vi "Load Parameters From XML.vi"() -> (0 "error out":errorcluster, 2 "dynamic parameters":cluster{"Thumb":T1, "Middle":T1, "Index":T1}, 3 "kinematic parameters":T4)   [LabVIEW 2011, in "MF3.lvclass"]
uses:
  MF3.lvclass
  <vilib>/robotics/Kinematics/Link/Joint Type.ctl
  Controls/5-bar Side.ctl
  Controls/Dynamic Parameters.ctl
  <vilib>/NI/GXML/_subVIs/GXML SearchParser/Search Parser.vi
  <vilib>/NI/GXML/GXML.lvlib
  <vilib>/robotics/Kinematics/Link/NI_Robotics_Link.lvclass
panel:
  out "file path":path
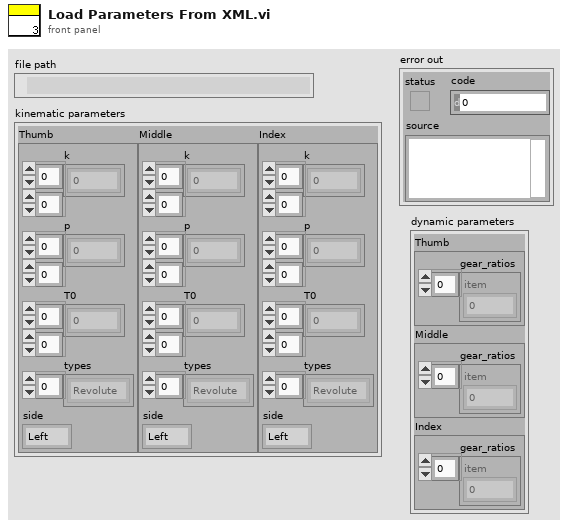
[diagram p1: front panel]
types:
  T1 = typedef "Dynamic Parameters.ctl" = cluster{"gear_ratios":sgl[]}
  T2 = typedef "NI_Robotics_Link.lvclass/Joint Type.ctl" = enum16{"Revolute", "Prismatic"}
  T3 = typedef "5-bar Side.ctl" = enum16{"Left", "Right"}
  T4 = cluster{"Thumb":cluster{"k":sgl[][], "p":sgl[][], "T0":sgl[][], "types":T2[], "side":T3}, "Middle":cluster{"k":sgl[][], "p":sgl[][], "T0":sgl[][], "types":T2[], "side":T3}, "Index":cluster{"k":sgl[][], "p":sgl[][], "T0":sgl[][], "types":T2[], "side":T3}}
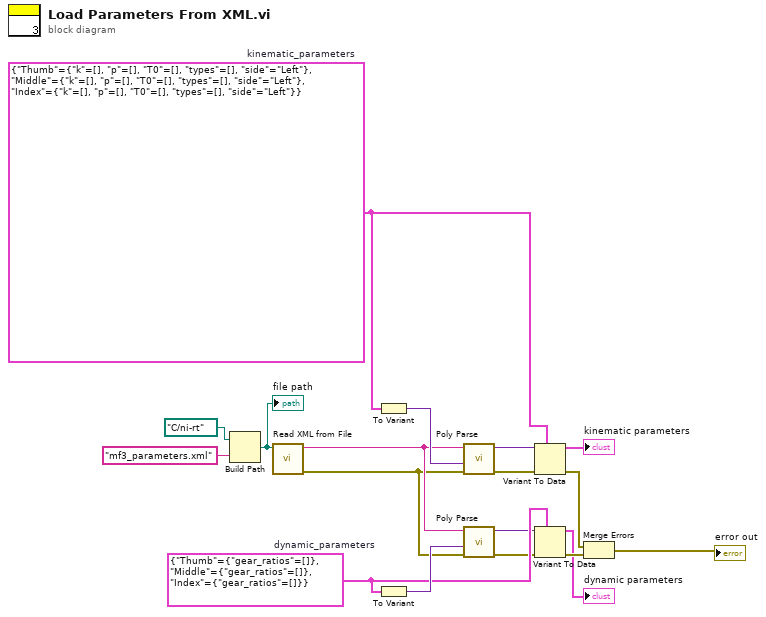
[diagram p0: block diagram]
diagram:
  w6 = cluster{"Thumb":T1, "Middle":T1, "Index":T1} {"Thumb"={"gear_ratios"=[]}, "Middle"={"gear_ratios"=[]}, "Index"={"gear_ratios"=[]}}  # dynamic_parameters
  w13 = T4 {"Thumb"={"k"=[], "p"=[], "T0"=[], "types"=[], "side"=enum."Left"}, "Middle"={"k"=[], "p"=[], "T0"=[], "types"=[], "side"=enum."Left"}, "Index"={"k"=[], "p"=[], "T0"=[], "types"=[], "side"=enum."Left"}}  # kinematic_parameters
  n1 = Build Path(base path=path "C:/ni-rt", name or relative path="mf3_parameters.xml") -> (appended path=w16:path)
  "file path" <- w16
  n2 = call <vilib>:"Read XML from File.vi"("XML File Path"=w16) -> ("error out"=w9:errorcluster, "XML String Out"=w10:string)  [unwired: 9 in]
  n3 = To Variant(anything=w13) -> (Variant=w15:variant)
  n4 = To Variant(anything=w6) -> (Variant=w11:variant)
  n5 = call-poly <vilib>:"Poly Parse.vi"("error in"=w9, "TypeDesc"=w15, "XML String In"=w10) -> ("error out"=w8:errorcluster, "Parsed Data"=w14:variant)  [unwired: 7 in]
  n6 = call-poly <vilib>:"Poly Parse.vi"("error in"=w9, "TypeDesc"=w11, "XML String In"=w10) -> ("error out"=w4:errorcluster, "Parsed Data"=w5:variant)  [unwired: 7 in]
  n7 = Variant To Data(error in=w8, type=w13, Variant=w14) -> (data=→"kinematic parameters":T4, error out=w7:errorcluster)
  n8 = Variant To Data(error in=w4, type=w6, Variant=w5) -> (data=→"dynamic parameters":cluster{"Thumb":T1, "Middle":T1, "Index":T1}, error out=w3:errorcluster)
  n9 = Merge Errors(w7, w3) -> (→"error out":errorcluster)
